vi "Aggiungi grafico.vi"(0 "Grafici":T1[](array[typedef]) {"ASSE Y 5"."Decimali" min=0 max=6; "ASSE Y 4"."Decimali" min=0 max=6; "ASSE Y 3"."Decimali" min=0 max=6; "ASSE Y 2"."Decimali" min=0 max=6; "ASSE Y 1"."Decimali" min=0 max=6; "ASSE X 2"."Decimali" min=0 max=6; "ASSE X 1"."Decimali" min=0 max=6}, 1 "Array plot":T9[](array[typedef]) {"PLOT"."GRANDEZZA Y" items=["Banco", "Anno", "Numero", "N° tabella", "Misura", "Tipo prova", "Progressivo Acq", "tempo[h:m:s]", "tempo acq[min]", "f [Hz]", "Uav [V]", "Iav [A]", "Tq [Nm]", "n [rpm]", "P1 [kW]", "P1 n[kW]", "Q [m3/h]", "Q n[m3/h]", "Q [l/min]", "Q n[l/min]", "H1 [m]", "Dislivello [m]", "Hdinamica [m]", "HvAsp [m]", "HvMand [m]", "HvTot [m]", "H2 [m]", "Htot [m]", "Htot n[m]", "P3 (Phyd) [kW]", "P3 (Phyd) n[kW]", "P2 [kW]", "P2 n[kW]", "P2 n ps[kW]", "eta motore [%]", "eta pompa [%]", "eta pompa n[%]", "eta gruppo [%]", "eta gruppo n[%]", "T acqua [°C]", "Densità liquido [kg/m3]", "P barometrica [mbar]", "pf", "Uch1 [V]", "Uch2 [V]", "Uch3 [V]", "Ich1 [A]", "Ich2 [A]", "Ich3 [A]", "Temp.amb[°C]", "Ru-w [ohm]", "DTavvolg. [°C]", "Tamb Freddo [°C]", "Ru-w Freddo [ohm]", "Tc1[°C]", "Tc2[°C]", "Tc3[°C]", "Tc4[°C]", "Tc5", "Tc6", "Tc7", "Tc8", "H1[Bar]", "H2[bar]", "P premist.[Bar]", "Pserb[bar]", "n°NPSH", "NPSH", "Htot Ref[m]", "NPSH_%caduta", "%caduta", "Qref [m3/h]", "MEI"]; "PLOT"."GRANDEZZA X" items=["Banco", "Anno", "Numero", "N° tabella", "Misura", "Tipo prova", "Progressivo Acq", "tempo[h:m:s]", "tempo acq[min]", "f [Hz]", "Uav [V]", "Iav [A]", "Tq [Nm]", "n [rpm]", "P1 [kW]", "P1 n[kW]", "Q [m3/h]", "Q n[m3/h]", "Q [l/min]", "Q n[l/min]", "H1 [m]", "Dislivello [m]", "Hdinamica [m]", "HvAsp [m]", "HvMand [m]", "HvTot [m]", "H2 [m]", "Htot [m]", "Htot n[m]", "P3 (Phyd) [kW]", "P3 (Phyd) n[kW]", "P2 [kW]", "P2 n[kW]", "P2 n ps[kW]", "eta motore [%]", "eta pompa [%]", "eta pompa n[%]", "eta gruppo [%]", "eta gruppo n[%]", "T acqua [°C]", "Densità liquido [kg/m3]", "P barometrica [mbar]", "pf", "Uch1 [V]", "Uch2 [V]", "Uch3 [V]", "Ich1 [A]", "Ich2 [A]", "Ich3 [A]", "Temp.amb[°C]", "Ru-w [ohm]", "DTavvolg. [°C]", "Tamb Freddo [°C]", "Ru-w Freddo [ohm]", "Tc1[°C]", "Tc2[°C]", "Tc3[°C]", "Tc4[°C]", "Tc5", "Tc6", "Tc7", "Tc8", "H1[Bar]", "H2[bar]", "P premist.[Bar]", "Pserb[bar]", "n°NPSH", "NPSH", "Htot Ref[m]", "NPSH_%caduta", "%caduta", "Qref [m3/h]", "MEI"]; "Assi grafico"."ASSE X" items=["X 1", "X 2"]; "Assi grafico"."ASSE Y" items=["Y 1", "Y 2", "Y 3", "Y 4"]}, 2 "Grafici":string[](array[string]), 3 "Grafico default":u16(ring), 4 "prova":i32, 5 "ID collegamenti":i32[](array[numeric]), 6 "Collaudi":string[](array[string]), 7 "Dati collaudo in corso":T8, 8 "AUTO":bool, 9 "Collaudi di confronto":T8[](array[typedef])) -> (14 "Image Data":T7, 15 "grafico":u16, 16 "Control descriptors out":T3, 17 "grafico.Text":string, 18 "annulla?":bool)   [LabVIEW 2019]
uses:
  TypeDef/Definizione_Grafico_REPORT.ctl
  TypeDef/Definizione_plot.ctl
  TypeDef/Dati collaudo.ctl
  <vilib>/picture/picture.llb/imagedata.ctl
  <userlib>/PropSaver/ps-TypeDefs.llb/[pstype] Array of Control's properties.ctl
  <userlib>/PropSaver/ps-TypeDefs.llb/[pstype] Control's Properties descriptor.ctl
  <userlib>/PropSaver/ps-TypeDefs.llb/[pstype] Array of Property descriptors.ctl
  <userlib>/PropSaver/ps-TypeDefs.llb/[pstype] Property descriptor.ctl
panel:
  in  "annulla":bool
  in  "GRAFICO":T1 {"ASSE Y 5"."Decimali" min=0 max=6; "ASSE Y 4"."Decimali" min=0 max=6; "ASSE Y 3"."Decimali" min=0 max=6; "ASSE Y 2"."Decimali" min=0 max=6; "ASSE Y 1"."Decimali" min=0 max=6; "ASSE X 2"."Decimali" min=0 max=6; "ASSE X 1"."Decimali" min=0 max=6}
  in  "Cluster":T2
  out "Numeric":i32
  in  "stop":bool
  out "GRAFICO GRANDE 1":cluster{"X":dbl[], "Y":dbl[]}[](graph)
  in  "Interpola?":cluster{"interpola?":bool, "order":dbl}[](array[cluster])=[{"interpola?"=FALSE, "order"=2.0}, {"interpola?"=FALSE, "order"=2.0}, {"interpola?"=FALSE, "order"=2.0}, {"interpola?"=FALSE, "order"=2.0}, {"interpola?"=FALSE, "order"=2.0}, {"interpola?"=FALSE, "order"=2.0}, {"interpola?"=FALSE, "order"=2.0}, {"interpola?"=FALSE, "order"=2.0}, {"interpola?"=FALSE, "order"=2.0}, {"interpola?"=FALSE, "order"=2.0}, {"interpola?"=FALSE, "order"=2.0}, {"interpola?"=FALSE, "order"=2.0}, {"interpola?"=FALSE, "order"=2.0}, {"interpola?"=FALSE, "order"=2.0}, {"interpola?"=FALSE, "order"=2.0}, {"interpola?"=FALSE, "order"=2.0}, {"interpola?"=FALSE, "order"=2.0}, {"interpola?"=FALSE, "order"=2.0}, {"interpola?"=FALSE, "order"=2.0}, {"interpola?"=FALSE, "order"=2.0}]
  in  "scelta grafico A VUOTO":u16(ring) items=["Test a Vuoto", "CosPhi"]
  # "SCELTA GRAFICO"
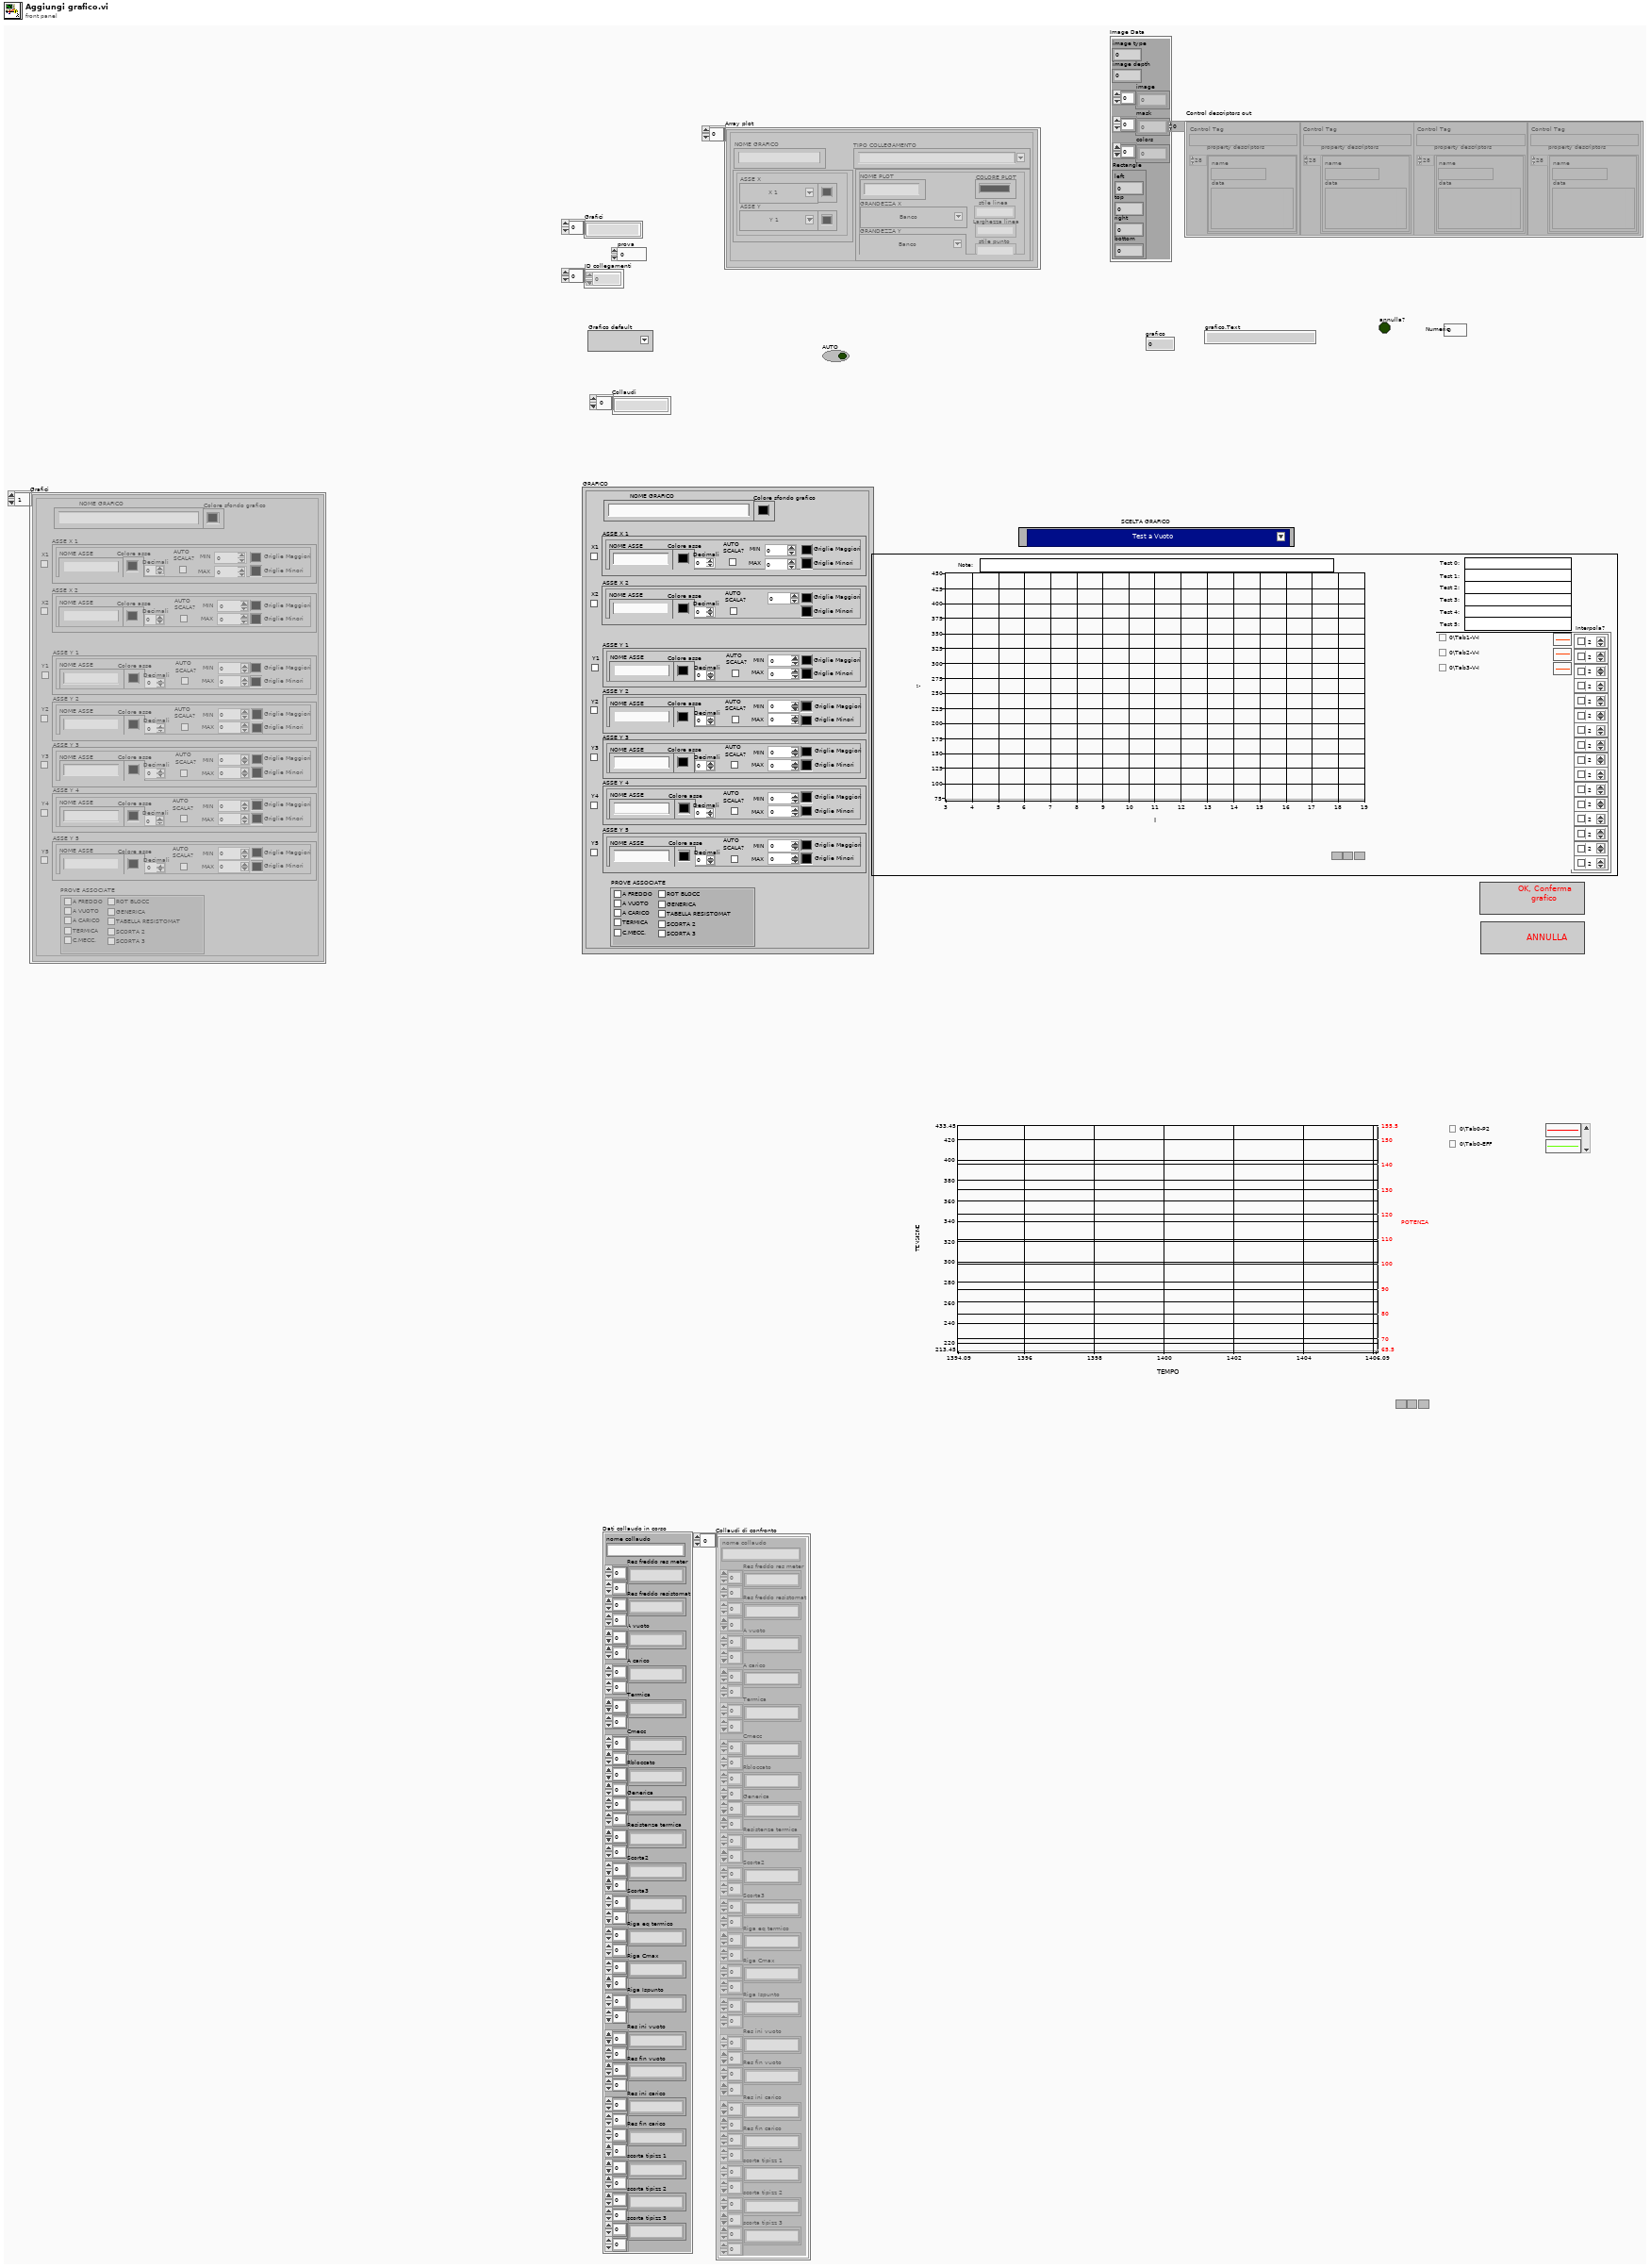
[diagram p1: front panel]
types:
  T1 = typedef "Definizione_Grafico_REPORT.ctl" = cluster{"ASSE X 1":cluster{"NOME ASSE":string, "AUTO\nSCALA?":bool, "MIN":dbl, "MAX":dbl, "Colore asse":u32, "Griglie Maggiori":u32, "Griglie Minori":u32, "Decimali":i8}, "ASSE X 2":cluster{"NOME ASSE":string, "AUTO\nSCALA?":bool, "MIN":dbl, "MAX":dbl, "Colore asse":u32, "Griglie Maggiori":u32, "Griglie Minori":u32, "Decimali":i8}, "ASSE Y 1":cluster{"NOME ASSE":string, "AUTO\nSCALA?":bool, "MIN":dbl, "MAX":dbl, "Colore asse":u32, "Griglie Maggiori":u32, "Griglie Minori":u32, "Decimali":i8}, "ASSE Y 2":cluster{"NOME ASSE":string, "AUTO\nSCALA?":bool, "MIN":dbl, "MAX":dbl, "Colore asse":u32, "Griglie Maggiori":u32, "Griglie Minori":u32, "Decimali":i8}, "ASSE Y 3":cluster{"NOME ASSE":string, "AUTO\nSCALA?":bool, "MIN":dbl, "MAX":dbl, "Colore asse":u32, "Griglie Maggiori":u32, "Griglie Minori":u32, "Decimali":i8}, "ASSE Y 4":cluster{"NOME ASSE":string, "AUTO\nSCALA?":bool, "MIN":dbl, "MAX":dbl, "Colore asse":u32, "Griglie Maggiori":u32, "Griglie Minori":u32, "Decimali":i8}, "X1":bool, "X2":bool, "Y1":bool, "Y2":bool, "Y3":bool, "Y4":bool, "NOME GRAFICO":string, "PROVE ASSOCIATE":cluster{"A FREDDO":bool, "A VUOTO":bool, "A CARICO":bool, "TERMICA":bool, "C.MECC.":bool, "ROT BLOCC":bool, "GENERICA":bool, "TABELLA RESISTOMAT":bool, "SCORTA 2":bool, "SCORTA 3":bool}, "ASSE Y 5":cluster{"NOME ASSE":string, "AUTO\nSCALA?":bool, "MIN":dbl, "MAX":dbl, "Colore asse":u32, "Griglie Maggiori":u32, "Griglie Minori":u32, "Decimali":i8}, "Y5":bool, "Colore sfondo grafico":u32}
  T2 = cluster{"GRAFICO GRANDE 1":cluster{"X":dbl[], "Y":dbl[]}[], "Note:":string, "Test 0:":string, "Test 1:":string, "Test 2:":string, "Test 3:":string, "Test 4:":string, "Test 5:":string}
  T3 = typedef "[pstype] Array of Control's properties.ctl" = T4[]
  T4 = typedef "[pstype] Control's Properties descriptor.ctl" = cluster{"Control Tag":string, "property descriptors":T5}
  T5 = typedef "[pstype] Array of Property descriptors.ctl" = T6[]
  T6 = typedef "[pstype] Property descriptor.ctl" = cluster{"name":string, "data":variant}
  T7 = typedef "imagedata.ctl" = cluster{"image type":i32, "image depth":i32, "image":u8[], "mask":u8[], "colors":u32[], "Rectangle":cluster{"left":i16, "top":i16, "right":i16, "bottom":i16}}
  T8 = typedef "Dati collaudo.ctl" = cluster{"nome collaudo":string, "Res freddo res meter":string[][], "Res freddo resistomat":string[][], "A vuoto":string[][], "A carico":string[][], "Termica":string[][], "Cmecc":string[][], "Rbloccato":string[][], "Generica":string[][], "Resistenze termica":string[][], "Scorta2":string[][], "Scorta3":string[][], "Riga eq termico":string[][], "Riga Cmax":string[][], "Riga Ispunto":string[][], "Res ini vuoto":string[][], "Res fin vuoto":string[][], "Res ini carico":string[][], "Res fin carico":string[][], "scorta tipizz 1":string[][], "scorta tipizz 2":string[][], "scorta tipizz 3":string[][]}
  T9 = typedef "Definizione_plot.ctl" = cluster{"Assi grafico":cluster{"ASSE Y":u16, "ASSE X":u16, "Colore x":u32, "Colore y":u32}, "TIPO COLLEGAMENTO":string, "PLOT":cluster{"GRANDEZZA X":u16, "GRANDEZZA Y":u16, "COLORE PLOT":u32, "NOME PLOT":string, "Larghezza linea":u16, "stile linea":u16, "stile punto":u16}, "NOME GRAFICO":string}
  T10 = enum32{"Invalid", "Standard", "Closed", "Hidden", "Minimized", "Maximized"}
  T11 = enum16{"no default", "value", "properties", "value & properties"}
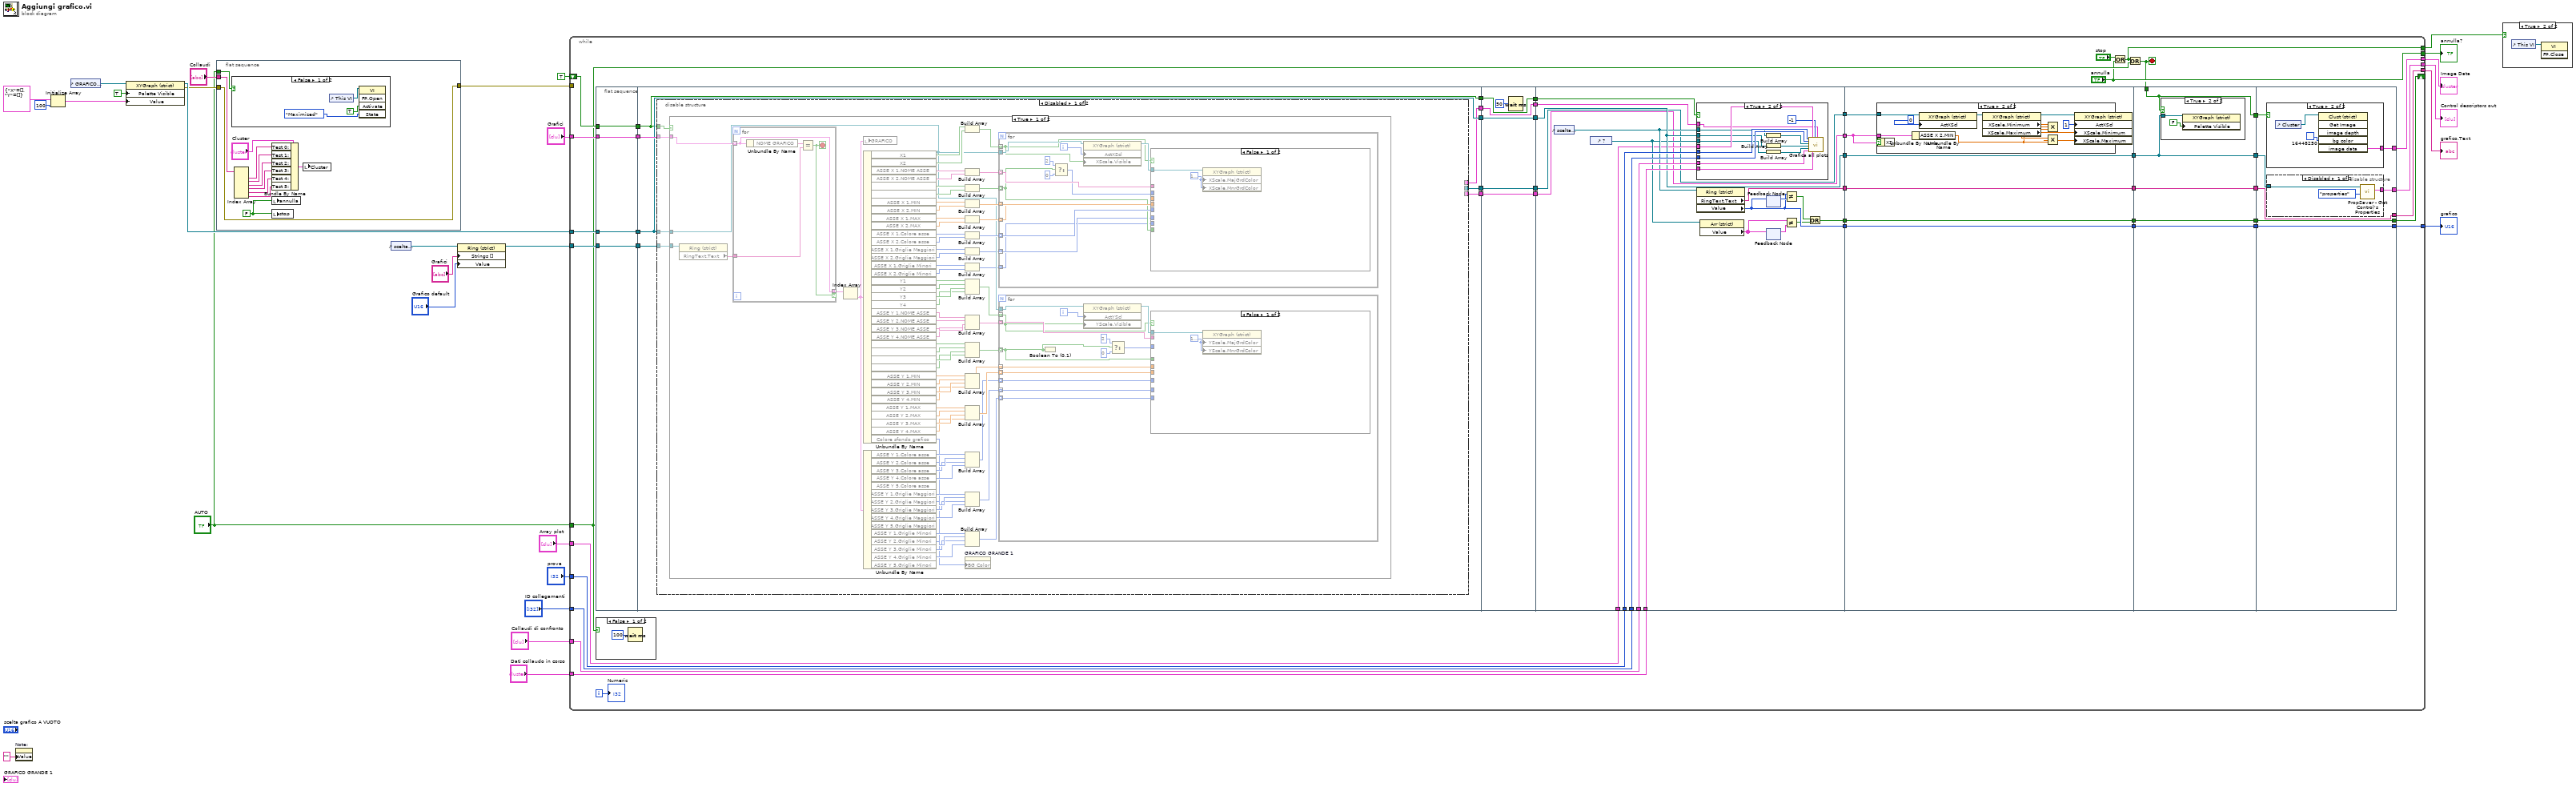
[diagram p0: block diagram]
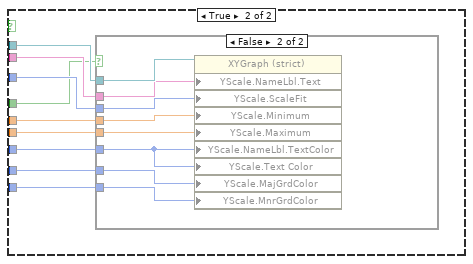
[diagram p5: hidden frame]
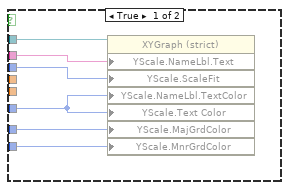
[diagram p6: hidden frame]
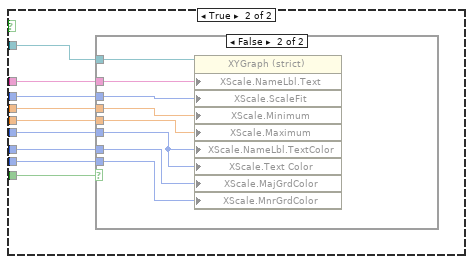
[diagram p7: hidden frame]
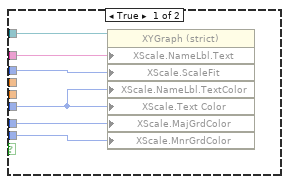
[diagram p8: hidden frame]
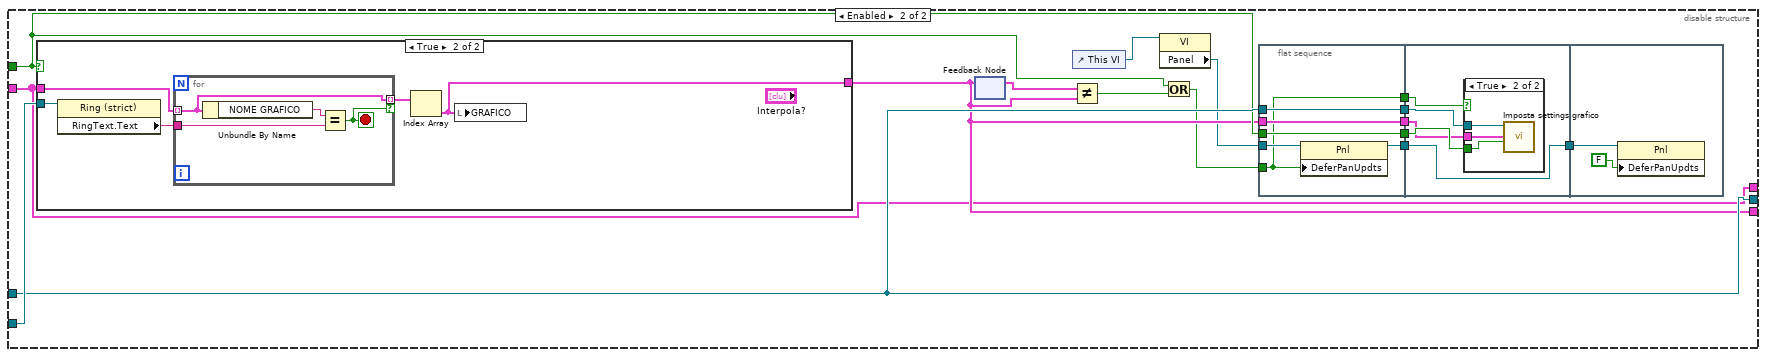
[diagram p10: hidden frame]
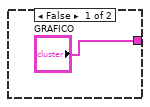
[diagram p12: hidden frame]
diagram:
  n1 = property on="Note:" class="Str"("Value"="") -> ()  [unwired: 2 in, 2 out]
  n2 = Initialize Array(cluster{"X":dbl[], "Y":dbl[]} {"X"=[], "Y"=[]} ("QP"), 100 ("dimension size")) -> (w6:cluster{"X":dbl[], "Y":dbl[]}[])
  n3 = control-ref of="GRAFICO GRANDE 1"() -> (w10:refnum<vi>)
  n4 = property class="XYGraph (strict)"(reference=w10, "Palette Visible"=TRUE ("Palette:Visible"), "Value"=w6) -> (reference out=w9:refnum<vi>, error out=w5:errorcluster)  [unwired: 1 in]
  n5 = flat-sequence {
    tunnel: w5 -> [w38]
    tunnel: [w38] -> w4
    tunnel: "Collaudi" -> [w37]
    tunnel: "AUTO" -> [w29]
    frame #0 {
      w30 = FALSE
      n6 = case shown="False" w29 {
        frame False {
          n7 = control-ref of="This VI"() -> (w43:refnum<vi>)
          n8 = invoke class="VI" method="FP.Open"(reference=w43, "Activate"=TRUE ("Activate?"), "State"=T10."Maximized") -> ()  [unwired: 2 in, 5 out]
        }
        frame True {
        }
      }
      n9 = Index Array(array=w37) -> (element #1=w36:string, element #2=w35:string, element #3=w34:string, element #4=w33:string, element #5=w32:string, element #6=w31:string)  [unwired: 6 in]
      n10 = Bundle By Name(cluster="Cluster", "Test 0:"=w36, "Test 1:"=w35, "Test 2:"=w34, "Test 3:"=w33, "Test 4:"=w32, "Test 5:"=w31) -> (w39:T2)
      n11 = local write "annulla"(w30) -> ()
      n12 = local write "stop"(w30) -> ()
      n13 = local write "Cluster"(w39) -> ()
    }
  }
  n14 = control-ref of="scelta grafico A VUOTO"() -> (w27:refnum<vi>)
  n15 = property class="Ring (strict)"(reference=w27, "Strings []"="Grafici", "Value"="Grafico default") -> (reference out=w26:refnum<vi>)  [unwired: 1 in, 1 out]
  n16 = while {
    tunnel: "Grafici" -> [w89]
    tunnel: w26 -> [w88]
    tunnel: "Array plot" -> [w87]
    tunnel: "prova" -> [w86]
    tunnel: "ID collegamenti" -> [w85]
    tunnel: "Dati collaudo in corso" -> [w84]
    tunnel: "Collaudi di confronto" -> [w83]
    tunnel: [w82] -> w20
    tunnel: w9 -> [w81]
    shift-right: [w80] -> _
    shift-left: TRUE -> [w78]
    tunnel: [w77] -> w18
    tunnel: [w76] -> w17
    tunnel: "AUTO" -> [w75]
    tunnel: [w49] -> w16
    tunnel: [w69] -> w15
    tunnel: w4 -> [_]
    tunnel: ["annulla"] -> w2
    i -> [w70]
    stop <- w47 stop-if-true
    n17 = flat-sequence {
      tunnel: w89 -> [w95]
      tunnel: w81 -> [w96]
      tunnel: w88 -> [w97]
      tunnel: [w97] -> w92
      tunnel: [w96] -> w91
      tunnel: [w95] -> w90
      tunnel: [w94] -> w79
      tunnel: w78 -> [w94]
      tunnel: [w102] -> w74
      tunnel: w92 -> [w104]
      tunnel: w91 -> [w102]
      tunnel: w90 -> [w103]
      tunnel: w79 -> [w101]
      tunnel: [w101] -> w71
      tunnel: [w100] -> w54
      tunnel: [w99] -> w51
      tunnel: [w98] -> w45
      tunnel: w74 -> [w310]
      tunnel: [w310] -> w73
      tunnel: [w309] -> w72
      tunnel: w71 -> [w309]
      tunnel: [w308] -> w55
      tunnel: w54 -> [w308]
      tunnel: [w307] -> w52
      tunnel: w51 -> [w307]
      tunnel: w45 -> [w305]
      tunnel: [w305] -> w44
      tunnel: w87 -> [w315]
      tunnel: w86 -> [w330]
      tunnel: w85 -> [w329]
      tunnel: w84 -> [w328]
      tunnel: w83 -> [w327]
      tunnel: [w326] -> w64
      tunnel: w73 -> [w326]
      tunnel: [w318] -> w62
      tunnel: [w322] -> w60
      tunnel: w72 -> [w316]
      tunnel: [w314] -> w58
      tunnel: [w313] -> w56
      tunnel: w55 -> [w313]
      tunnel: [w312] -> w53
      tunnel: w52 -> [w312]
      tunnel: w44 -> [w311]
      tunnel: w64 -> [w350]
      tunnel: [w350] -> w63
      tunnel: w62 -> [w349]
      tunnel: [w349] -> w61
      tunnel: w60 -> [w348]
      tunnel: [w348] -> w59
      tunnel: w58 -> [w347]
      tunnel: [w347] -> w57
      tunnel: w56 -> [w345]
      tunnel: w53 -> [w344]
      tunnel: w63 -> [w363]
      tunnel: [w363] -> w68
      tunnel: w61 -> [w366]
      tunnel: [w366] -> w67
      tunnel: w59 -> [w365]
      tunnel: [w365] -> w66
      tunnel: w57 -> [w364]
      tunnel: [w364] -> w65
      tunnel: w47 -> [w362]
      tunnel: [w362] -> w46
      tunnel: w68 -> [w372]
      tunnel: [w375] -> w82
      tunnel: [w374] -> w80
      tunnel: w67 -> [w374]
      tunnel: [w373] -> w77
      tunnel: w66 -> [w373]
      tunnel: [w371] -> w76
      tunnel: [w370] -> w69
      tunnel: w65 -> [w370]
      tunnel: w46 -> [w369]
      frame #0 {
      }
      frame #1 {
        n18 = disable-structure shown="Disabled" {
          disable-tunnel: w104 -> [w108 w278]
          disable-tunnel: w103 -> [w107 w263]
          disable-tunnel: w102 -> [w106 w277]
          disable-tunnel: w101 -> [w105 w276]
          disable-tunnel: [_ w274] -> w100
          disable-tunnel: [_ w277] -> w99
          disable-tunnel: [_ w263] -> w98
          frame Disabled {
            n19 = case shown="True" w105 {
              tunnel: w108 -> [w179 _]
              tunnel: w107 -> [w135 _]
              tunnel: w106 -> [w134 w262]
              frame True {
                n20 = property class="Ring (strict)"(reference=w179) -> ("RingText.Text"=w178:string)  [unwired: 1 in, 2 out]
                n21 = for {
                  tunnel: w135 -> [w261] mode=indexing
                  tunnel: w178 -> [w259]
                  tunnel: [w261] -> w177 mode=indexing if=w258
                  stop <- w258 stop-if-true
                  n22 = Unbundle By Name(w261) -> ("NOME GRAFICO"=w260:string)
                  n23 = Equal?(x=w260, y=w259) -> (x = y?=w258:bool)
                }
                n24 = Index Array(array=w177) -> (element=w109:T1)  [unwired: 1 in]
                n25 = local write "GRAFICO"(w109) -> ()
                n26 = Unbundle By Name(w109) -> ("X1"=w176:bool, "X2"=w175:bool, "ASSE X 1.NOME ASSE"=w173:string, "ASSE X 2.NOME ASSE"=w149:string, "ASSE X 1.AUTO\nSCALA?"=w148:bool, "ASSE X 2.AUTO\nSCALA?"=w147:bool, "ASSE X 1.MIN"=w146:dbl, "ASSE X 2.MIN"=w145:dbl, "ASSE X 1.MAX"=w144:dbl, "ASSE X 2.MAX"=w143:dbl, "ASSE X 1.Colore asse"=w129:u32, "ASSE X 2.Colore asse"=w128:u32, "ASSE X 1.Griglie Maggiori"=w126:u32, "ASSE X 2.Griglie Maggiori"=w125:u32, "ASSE X 1.Griglie Minori"=w123:u32, "ASSE X 2.Griglie Minori"=w122:u32, "Y1"=w127:bool, "Y2"=w168:bool, "Y3"=w167:bool, "Y4"=w166:bool, "ASSE Y 1.NOME ASSE"=w165:string, "ASSE Y 2.NOME ASSE"=w164:string, "ASSE Y 3.NOME ASSE"=w163:string, "ASSE Y 4.NOME ASSE"=w162:string, "ASSE Y 1.AUTO\nSCALA?"=w161:bool, "ASSE Y 2.AUTO\nSCALA?"=w160:bool, "ASSE Y 3.AUTO\nSCALA?"=w159:bool, "ASSE Y 4.AUTO\nSCALA?"=w158:bool, "ASSE Y 1.MIN"=w157:dbl, "ASSE Y 2.MIN"=w156:dbl, "ASSE Y 3.MIN"=w155:dbl, "ASSE Y 4.MIN"=w154:dbl, "ASSE Y 1.MAX"=w153:dbl, "ASSE Y 2.MAX"=w152:dbl, "ASSE Y 3.MAX"=w151:dbl, "ASSE Y 4.MAX"=w150:dbl, "Colore sfondo grafico"=w110:u32)
                n27 = Unbundle By Name(w109) -> ("ASSE Y 1.Colore asse"=w133:u32, "ASSE Y 2.Colore asse"=w132:u32, "ASSE Y 3.Colore asse"=w131:u32, "ASSE Y 4.Colore asse"=w130:u32, "ASSE Y 1.Griglie Maggiori"=w120:u32, "ASSE Y 2.Griglie Maggiori"=w119:u32, "ASSE Y 3.Griglie Maggiori"=w118:u32, "ASSE Y 4.Griglie Maggiori"=w117:u32, "ASSE Y 1.Griglie Minori"=w115:u32, "ASSE Y 2.Griglie Minori"=w114:u32, "ASSE Y 3.Griglie Minori"=w113:u32, "ASSE Y 4.Griglie Minori"=w112:u32)  [unwired: 3 out]
                n28 = Build Array(w176, w175) -> (w174:bool[])
                n29 = Build Array(w173, w149) -> (w172:string[])
                n30 = Build Array(w148, w147) -> (w171:bool[])
                n31 = Build Array(w146, w145) -> (w170:dbl[])
                n32 = Build Array(w144, w143) -> (w169:dbl[])
                n33 = Build Array(w129, w128) -> (w137:u32[])
                n34 = Build Array(w126, w125) -> (w124:u32[])
                n35 = Build Array(w123, w122) -> (w121:u32[])
                n36 = Build Array(w127, w168, w167, w166) -> (w142:bool[])
                n37 = Build Array(w165, w164, w163, w162) -> (w141:string[])
                n38 = Build Array(w161, w160, w159, w158) -> (w140:bool[])
                n39 = Build Array(w157, w156, w155, w154) -> (w139:dbl[])
                n40 = Build Array(w153, w152, w151, w150) -> (w138:dbl[])
                n41 = Build Array(w133, w132, w131, w130) -> (w136:u32[])
                n42 = Build Array(w120, w119, w118, w117) -> (w116:u32[])
                n43 = Build Array(w115, w114, w113, w112) -> (w111:u32[])
                n44 = property on="GRAFICO GRANDE 1" class="XYGraph (strict)"("BG Color"=w110) -> ()  [unwired: 2 in, 2 out]
                n45 = for {
                  tunnel: w174 -> [w226] mode=indexing
                  tunnel: w134 -> [w232]
                  tunnel: w172 -> [w229] mode=indexing
                  tunnel: w171 -> [w221] mode=indexing
                  tunnel: w170 -> [w228] mode=indexing
                  tunnel: w169 -> [w227] mode=indexing
                  tunnel: w137 -> [w225] mode=indexing
                  tunnel: w124 -> [w220] mode=indexing
                  tunnel: w121 -> [w219] mode=indexing
                  i -> [w231]
                  n46 = Select(t=i16 2 ("0, 1"), s=w221, f=i16 0 ("0, 1")) -> (s? t:f=w222:i16)
                  n47 = property class="XYGraph (strict)"(reference=w232, "ActXScl"=w231, "XScale.Visible"=w226) -> (reference out=w230:refnum<vi>)  [unwired: 1 in, 1 out]
                  n48 = case shown="False" w226 {
                    tunnel: w230 -> [w234 w243]
                    tunnel: w229 -> [_ w242]
                    tunnel: w222 -> [_ w241]
                    tunnel: w228 -> [_ w240]
                    tunnel: w227 -> [_ w239]
                    tunnel: w225 -> [_ w238]
                    tunnel: w221 -> [_ w237]
                    tunnel: w220 -> [_ w236]
                    tunnel: w219 -> [_ w235]
                    frame False {
                      w233 = u32 16777216
                      n49 = property class="XYGraph (strict)"(reference=w234, "XScale.MajGrdColor"=w233, "XScale.MnrGrdColor"=w233) -> ()  [unwired: 1 in, 2 out]
                    }
                    frame True {
                      n50 = case shown="False" w237 {
                        tunnel: w243 -> [w249 w257]
                        tunnel: w242 -> [w248 w256]
                        tunnel: w241 -> [w247 w255]
                        tunnel: w240 -> [_ w254]
                        tunnel: w239 -> [_ w253]
                        tunnel: w238 -> [w246 w252]
                        tunnel: w236 -> [w245 w251]
                        tunnel: w235 -> [w244 w250]
                        frame True {
                          n51 = property class="XYGraph (strict)"(reference=w249, "XScale.NameLbl.Text"=w248, "XScale.ScaleFit"=w247, "XScale.NameLbl.TextColor"=w246, "XScale.Text Color"=w246, "XScale.MajGrdColor"=w245, "XScale.MnrGrdColor"=w244) -> ()  [unwired: 1 in, 2 out]
                        }
                        frame False {
                          n52 = property class="XYGraph (strict)"(reference=w257, "XScale.NameLbl.Text"=w256, "XScale.ScaleFit"=w255, "XScale.Minimum"=w254, "XScale.Maximum"=w253, "XScale.NameLbl.TextColor"=w252, "XScale.Text Color"=w252, "XScale.MajGrdColor"=w251, "XScale.MnrGrdColor"=w250) -> ()  [unwired: 1 in, 2 out]
                        }
                      }
                    }
                  }
                }
                n53 = for {
                  tunnel: w142 -> [w187] mode=indexing
                  tunnel: w134 -> [w193]
                  tunnel: w141 -> [w190] mode=indexing
                  tunnel: w140 -> [w182] mode=indexing
                  tunnel: w139 -> [w189] mode=indexing
                  tunnel: w138 -> [w188] mode=indexing
                  tunnel: w136 -> [w186] mode=indexing
                  tunnel: w116 -> [w181] mode=indexing
                  tunnel: w111 -> [w180] mode=indexing
                  i -> [w192]
                  n54 = Boolean To (0,1)(Boolean=w182) -> ()  [unwired: 1 out]
                  n55 = property class="XYGraph (strict)"(reference=w193, "ActYScl"=w192, "YScale.Visible"=w187) -> (reference out=w191:refnum<vi>)  [unwired: 1 in, 1 out]
                  n56 = Select(t=i16 2 ("0, 1"), s=w182, f=i16 0 ("0, 1")) -> (s? t:f=w183:i16)
                  n57 = case shown="False" w187 {
                    tunnel: w191 -> [w195 w204]
                    tunnel: w190 -> [_ w203]
                    tunnel: w183 -> [_ w202]
                    tunnel: w189 -> [_ w201]
                    tunnel: w188 -> [_ w200]
                    tunnel: w186 -> [_ w199]
                    tunnel: w182 -> [_ w198]
                    tunnel: w181 -> [_ w197]
                    tunnel: w180 -> [_ w196]
                    frame False {
                      w194 = u32 16777216
                      n58 = property class="XYGraph (strict)"(reference=w195, "YScale.MajGrdColor"=w194, "YScale.MnrGrdColor"=w194) -> ()  [unwired: 1 in, 2 out]
                    }
                    frame True {
                      n59 = case shown="False" w198 {
                        tunnel: w204 -> [w210 w218]
                        tunnel: w203 -> [w209 w217]
                        tunnel: w202 -> [w208 w216]
                        tunnel: w201 -> [_ w215]
                        tunnel: w200 -> [_ w214]
                        tunnel: w199 -> [w207 w213]
                        tunnel: w197 -> [w206 w212]
                        tunnel: w196 -> [w205 w211]
                        frame True {
                          n60 = property class="XYGraph (strict)"(reference=w210, "YScale.NameLbl.Text"=w209, "YScale.ScaleFit"=w208, "YScale.NameLbl.TextColor"=w207, "YScale.Text Color"=w207, "YScale.MajGrdColor"=w206, "YScale.MnrGrdColor"=w205) -> ()  [unwired: 1 in, 2 out]
                        }
                        frame False {
                          n61 = property class="XYGraph (strict)"(reference=w218, "YScale.NameLbl.Text"=w217, "YScale.ScaleFit"=w216, "YScale.Minimum"=w215, "YScale.Maximum"=w214, "YScale.NameLbl.TextColor"=w213, "YScale.Text Color"=w213, "YScale.MajGrdColor"=w212, "YScale.MnrGrdColor"=w211) -> ()  [unwired: 1 in, 2 out]
                        }
                      }
                    }
                  }
                }
              }
              frame False {
              }
            }
          }
          frame Enabled {
            n62 = case shown="True" w276 {
              tunnel: w263 -> [_ w298]
              tunnel: w278 -> [_ w297]
              tunnel: ["GRAFICO" w296] -> w274
              frame False {
              }
              frame True {
                n63 = property class="Ring (strict)"(reference=w297) -> ("RingText.Text"=w300:string)  [unwired: 1 in, 2 out]
                n64 = for {
                  tunnel: w298 -> [w304] mode=indexing
                  tunnel: w300 -> [w302]
                  tunnel: [w304] -> w299 mode=indexing if=w301
                  stop <- w301 stop-if-true
                  n65 = Unbundle By Name(w304) -> ("NOME GRAFICO"=w303:string)
                  n66 = Equal?(x=w303, y=w302) -> (x = y?=w301:bool)
                }
                n67 = Index Array(array=w299) -> (element=w296:T1)  [unwired: 1 in]
                n68 = local write "GRAFICO"(w296) -> ()
              }
            }
            n69 = feedback-in #1(w274) -> ()
            n70 = feedback #1() -> (w275:T1)  [unwired: 1 in]
            n71 = Not Equal?(x=w275, y=w274) -> (x != y?=w273:bool)
            n72 = control-ref of="This VI"() -> (w267:refnum<vi>)
            n73 = property class="VI"(reference=w267) -> ("Panel"=w266:refnum<vi>)  [unwired: 1 in, 2 out]
            n74 = Or(x=w276, y=w273) -> (x .or. y?=w272:bool)
            n75 = flat-sequence {
              tunnel: w272 -> [w280]
              tunnel: w274 -> [w282]
              tunnel: w276 -> [w283]
              tunnel: w277 -> [w284]
              tunnel: [w284] -> w271
              tunnel: [w283] -> w270
              tunnel: [w282] -> w269
              tunnel: [w280] -> w268
              tunnel: w266 -> [w281]
              tunnel: [w279] -> w264
              tunnel: w271 -> [w289]
              tunnel: w270 -> [w288]
              tunnel: w269 -> [w287]
              tunnel: w268 -> [w286]
              tunnel: [w285] -> w265
              tunnel: w264 -> [w285]
              tunnel: w265 -> [w294]
              frame #0 {
                n76 = property class="Pnl"(reference=w281, "DeferPanUpdts"=w280) -> (reference out=w279:refnum<vi>)  [unwired: 1 in, 1 out]
              }
              frame #1 {
                n77 = case shown="True" w286 {
                  tunnel: w289 -> [_ w292]
                  tunnel: w288 -> [_ w291]
                  tunnel: w287 -> [_ w290]
                  frame False {
                  }
                  frame True {
                    n78 = call "Imposta settings grafico.vi"("Reiniz nome plot"=w291, "GRAFICO"=w290, "XYGraph in"=w292) -> ()  [unwired: 9 in]
                  }
                }
              }
              frame #2 {
                n79 = property class="Pnl"(reference=w294, "DeferPanUpdts"=FALSE ("Defer Panel Updates")) -> ()  [unwired: 1 in, 2 out]
              }
            }
          }
        }
      }
      frame #2 {
        n80 = Wait (ms)(milliseconds to wait=u32 50) -> ()  [unwired: 1 out]
      }
      frame #3 {
        n81 = control-ref of="scelta grafico A VUOTO"() -> (w325:refnum<vi>)
        n82 = control-ref of="?"() -> (w321:refnum<vi>)
        n83 = case shown="True" w316 {
          tunnel: w315 -> [_ w343]
          tunnel: w330 -> [_ w342]
          tunnel: w329 -> [_ w341]
          tunnel: w328 -> [_ w340]
          tunnel: w327 -> [_ w339]
          tunnel: w326 -> [_ w338]
          tunnel: w325 -> [_ w334]
          tunnel: w321 -> [_ w333]
          tunnel: w311 -> [_ w331]
          frame False {
          }
          frame True {
            n84 = Build Array(w334) -> (w335:refnum<vi>[])
            n85 = Build Array(w338) -> (w336:refnum<vi>[])
            n86 = Build Array(w333) -> (w337:refnum<vi>[])
            n87 = call "Grafica all plots.vi"("prova"=w342, "ID COLLEGAMENTI"=w341, "Array scelte grafici"=w335, "Array Grafici"=w336, "array interpolazioni"=w337, "Collaudi di confronto"=w339, "Array plot"=w343, "Dati collaudo in corso"=w340, "Tabella in corso"=-1, "Grafici"=w331) -> ()  [unwired: 10 in]
          }
        }
        n88 = property class="Ring (strict)"(reference=w325) -> ("RingText.Text"=w314:string, "Value"=w322:u16)  [unwired: 1 in, 2 out]
        n89 = property class="Arr (strict)"(reference=w321) -> ("Value"=w319:cluster{"interpola?":bool, "order":dbl}[])  [unwired: 1 in, 2 out]
        n90 = feedback-in #2(w322) -> ()
        n91 = feedback #2() -> (w324:u16)  [unwired: 1 in]
        n92 = feedback #3() -> (w320:cluster{"interpola?":bool, "order":dbl}[])  [unwired: 1 in]
        n93 = feedback-in #3(w319) -> ()
        n94 = Not Equal?(x=w322, y=w324) -> (x != y?=w323:bool)
        n95 = Not Equal?(x=w319, y=w320) -> (x != y?=w317:bool)
        n96 = Or(x=w323, y=w317) -> (x .or. y?=w318:bool)
      }
      frame #4 {
        n97 = Unbundle By Name(w345) -> ("X2"=w346:bool)
        n98 = case shown="True" w346 {
          tunnel: w344 -> [_ w360]
          tunnel: w345 -> [_ w352]
          frame False {
          }
          frame True {
            n99 = Unbundle By Name(w352) -> ("ASSE X 2.MIN"=w351:dbl)
            n100 = property class="XYGraph (strict)"(reference=w360, "ActXScl"=0 ("Active X Scale")) -> (reference out=w358:refnum<vi>)  [unwired: 1 in, 1 out]
            n101 = property class="XYGraph (strict)"(reference=w358) -> (reference out=w357:refnum<vi>, "XScale.Minimum"=w356:dbl, "XScale.Maximum"=w354:dbl)  [unwired: 1 in, 1 out]
            n102 = Multiply(x=w356, y=w351) -> (x*y=w355:dbl)
            n103 = Multiply(x=w354, y=w351) -> (x*y=w353:dbl)
            n104 = property class="XYGraph (strict)"(reference=w357, "ActXScl"=1 ("Active X Scale"), "XScale.Minimum"=w355, "XScale.Maximum"=w353) -> ()  [unwired: 1 in, 2 out]
          }
        }
      }
      frame #5 {
        n105 = case shown="True" w362 {
          tunnel: w363 -> [_ w367]
          frame False {
          }
          frame True {
            n106 = property class="XYGraph (strict)"(reference=w367, "Palette Visible"=FALSE ("Palette:Visible")) -> ()  [unwired: 1 in, 2 out]
          }
        }
      }
      frame #6 {
        n107 = case shown="True" w369 {
          tunnel: [_ w377] -> w375
          frame False {
          }
          frame True {
            n108 = control-ref of="Cluster"() -> (w376:refnum<vi>)
            n109 = invoke class="Clust (strict)" method="Get Image"(reference=w376, "bg color"=u32 16448250) -> ("image data"=w377:T7)  [unwired: 4 in, 5 out]
          }
        }
        n110 = disable-structure shown="Disabled" {
          disable-tunnel: w372 -> [w381 _]
          disable-tunnel: [w380 _] -> w371
          frame Disabled {
            n111 = call <userlib>:"PropSaver - Get Control's Properties.vi"("get default (v&p)"=T11."properties", "Ctl Refnum"=w381) -> ("Control descriptors out"=w380:T3)  [unwired: 7 in, 2 out]
          }
          frame Enabled {
          }
        }
      }
    }
    n112 = case shown="False" w75 {
      frame False {
        n113 = Wait (ms)(milliseconds to wait=u32 100) -> ()  [unwired: 1 out]
      }
      frame True {
      }
    }
    n114 = Or(x="stop", y="annulla") -> (x .or. y?=w49:bool)
    n115 = Or(x=w49, y=w75) -> (x .or. y?=w47:bool)
    "Numeric" <- w70
  }
  "Image Data" <- w20
  "grafico" <- w18
  "Control descriptors out" <- w17
  "grafico.Text" <- w15
  "annulla?" <- w2
  n116 = case shown="True" w16 {
    frame False {
    }
    frame True {
      n117 = control-ref of="This VI"() -> (w382:refnum<vi>)
      n118 = invoke class="VI" method="FP.Close"(reference=w382) -> ()  [unwired: 2 in, 3 out]
    }
  }
